vi "glueing_proc_ORIG.vi"() -> ()   [LabVIEW 2011]
panel:
  in  "spint down 2":bool
  in  "glue press 2mm":bool
  in  "spint down":bool
  in  "Start":bool
  in  "fine tuning z dw 1mm":bool
  in  "fine tuning z up 1mm":bool
  in  "goto z pos 2":bool
  in  "goto z pos":bool
  in  "goto y pos":bool
  in  "positioning done":bool
  in  "goto x pos":bool
  in  "zero Spint":bool
  out "output":string
  out "command":string
  in  "zero done":bool
  in  "zero Gluer":bool
  in  "zero x":bool
  in  "zero y":bool
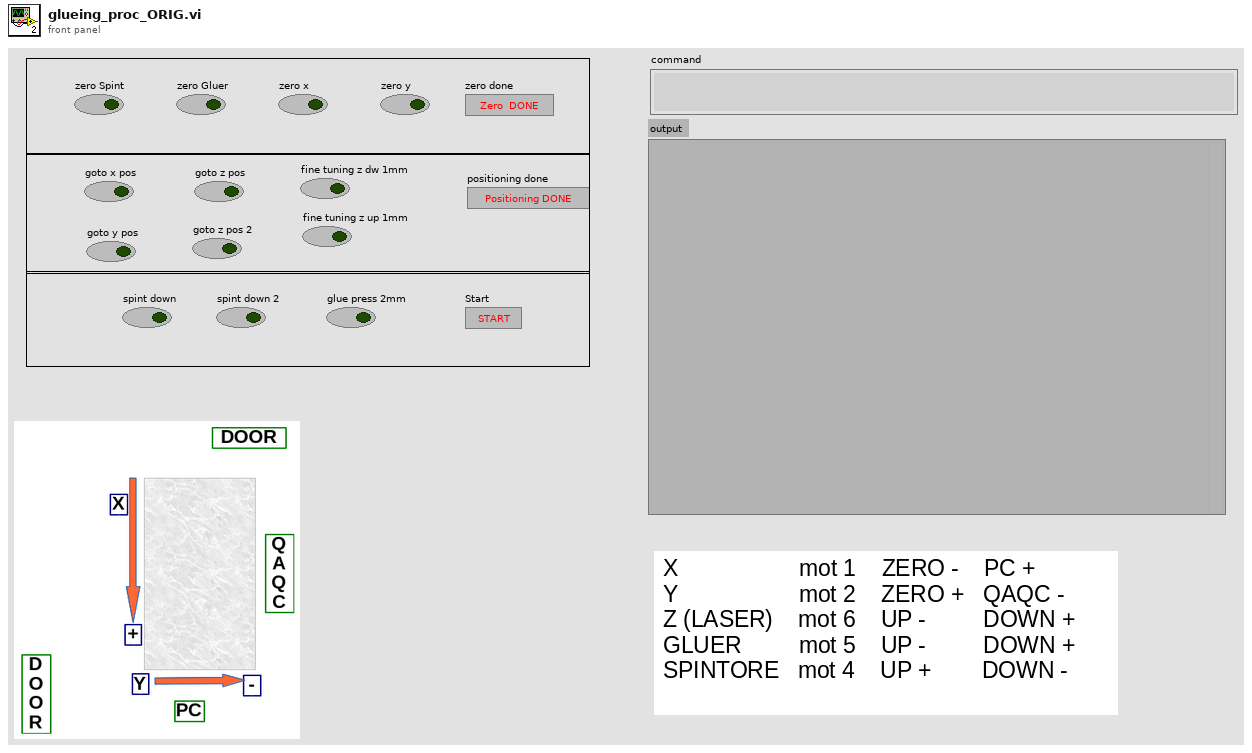
[diagram p1: front panel]
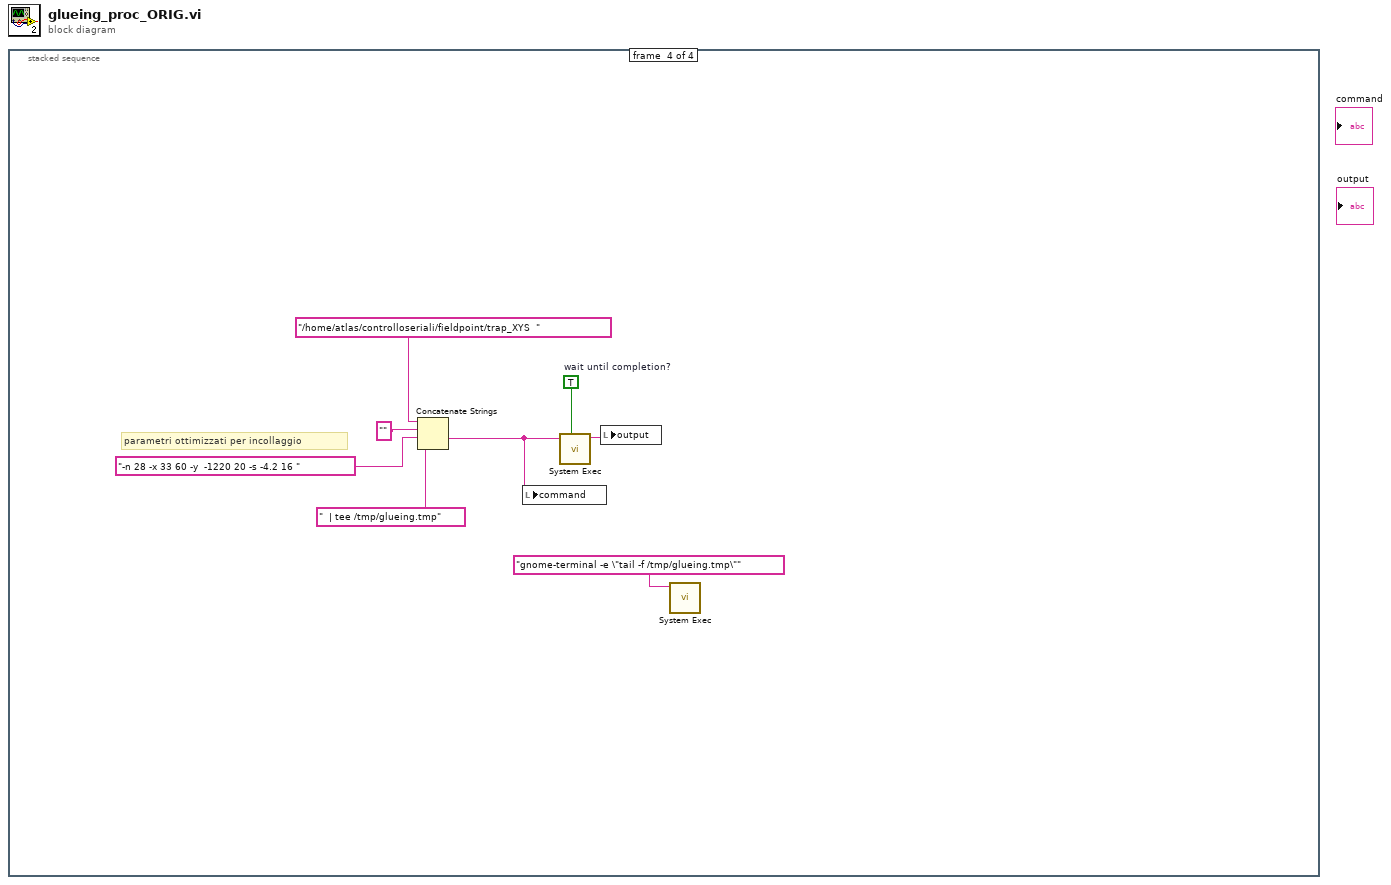
[diagram p0: block diagram]
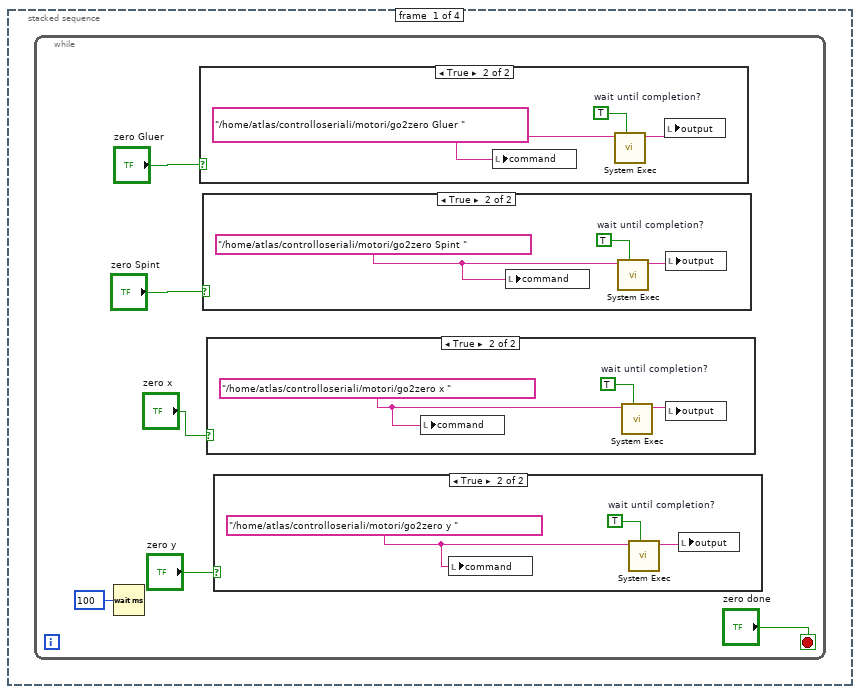
[diagram p2: hidden frame]
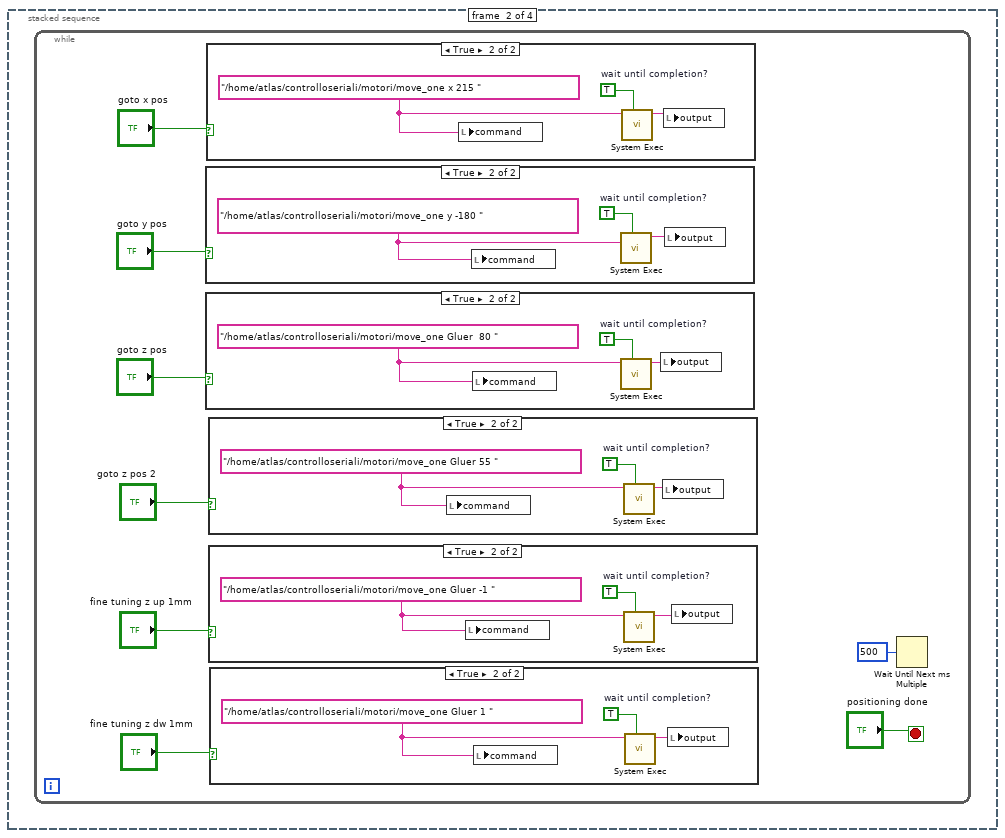
[diagram p7: hidden frame]
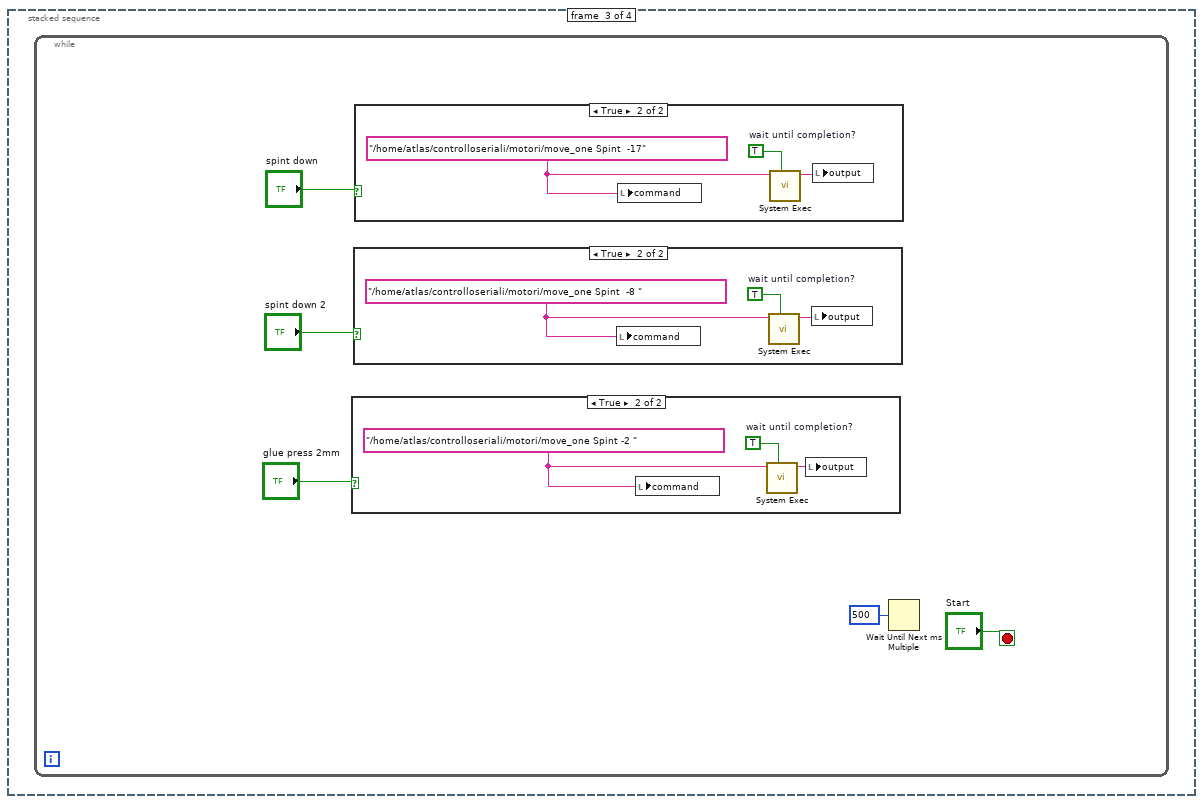
[diagram p14: hidden frame]
diagram:
  n1 = stacked-sequence {
    frame #0 {
      n2 = while {
        stop <- "zero done" stop-if-true
        n3 = Wait (ms)(milliseconds to wait=u32 100) -> ()  [unwired: 1 out]
        n4 = case shown="True" "zero Gluer" {
          frame False {
          }
          frame True {
            w17 = "/home/atlas/controlloseriali/motori/go2zero Gluer " ("string")
            w18 = TRUE  # wait until completion?
            n5 = local write "command"(w17) -> ()
            n6 = call <vilib>:"System Exec.vi"("wait until completion? (T)"=w18, "command line"=w17) -> ("standard output"=w16:string)  [unwired: 6 in, 3 out]
            n7 = local write "output"(w16) -> ()
          }
        }
        n8 = case shown="True" "zero Spint" {
          frame False {
          }
          frame True {
            w7 = "/home/atlas/controlloseriali/motori/go2zero Spint " ("string")
            w9 = TRUE  # wait until completion?
            n9 = local write "command"(w7) -> ()
            n10 = call <vilib>:"System Exec.vi"("wait until completion? (T)"=w9, "command line"=w7) -> ("standard output"=w8:string)  [unwired: 6 in, 3 out]
            n11 = local write "output"(w8) -> ()
          }
        }
        n12 = case shown="True" "zero x" {
          frame False {
          }
          frame True {
            w14 = "/home/atlas/controlloseriali/motori/go2zero x " ("string")
            w15 = TRUE  # wait until completion?
            n13 = local write "command"(w14) -> ()
            n14 = call <vilib>:"System Exec.vi"("wait until completion? (T)"=w15, "command line"=w14) -> ("standard output"=w13:string)  [unwired: 6 in, 3 out]
            n15 = local write "output"(w13) -> ()
          }
        }
        n16 = case shown="True" "zero y" {
          frame False {
          }
          frame True {
            w11 = "/home/atlas/controlloseriali/motori/go2zero y " ("string")
            w12 = TRUE  # wait until completion?
            n17 = local write "command"(w11) -> ()
            n18 = call <vilib>:"System Exec.vi"("wait until completion? (T)"=w12, "command line"=w11) -> ("standard output"=w10:string)  [unwired: 6 in, 3 out]
            n19 = local write "output"(w10) -> ()
          }
        }
      }
    }
    frame #1 {
      n20 = while {
        stop <- "positioning done" stop-if-true
        n21 = case shown="True" "goto y pos" {
          frame False {
          }
          frame True {
            w39 = "/home/atlas/controlloseriali/motori/move_one y -180 " ("string")
            w41 = TRUE  # wait until completion?
            n22 = local write "command"(w39) -> ()
            n23 = call <vilib>:"System Exec.vi"("wait until completion? (T)"=w41, "command line"=w39) -> ("standard output"=w40:string)  [unwired: 6 in, 3 out]
            n24 = local write "output"(w40) -> ()
          }
        }
        n25 = case shown="True" "goto z pos" {
          frame False {
          }
          frame True {
            w36 = "/home/atlas/controlloseriali/motori/move_one Gluer  80 " ("string")
            w38 = TRUE  # wait until completion?
            n26 = local write "command"(w36) -> ()
            n27 = call <vilib>:"System Exec.vi"("wait until completion? (T)"=w38, "command line"=w36) -> ("standard output"=w37:string)  [unwired: 6 in, 3 out]
            n28 = local write "output"(w37) -> ()
          }
        }
        n29 = case shown="True" "goto x pos" {
          frame False {
          }
          frame True {
            w42 = "/home/atlas/controlloseriali/motori/move_one x 215 " ("string")
            w44 = TRUE  # wait until completion?
            n30 = local write "command"(w42) -> ()
            n31 = call <vilib>:"System Exec.vi"("wait until completion? (T)"=w44, "command line"=w42) -> ("standard output"=w43:string)  [unwired: 6 in, 3 out]
            n32 = local write "output"(w43) -> ()
          }
        }
        n33 = case shown="True" "goto z pos 2" {
          frame False {
          }
          frame True {
            w33 = "/home/atlas/controlloseriali/motori/move_one Gluer 55 " ("string")
            w35 = TRUE  # wait until completion?
            n34 = local write "command"(w33) -> ()
            n35 = call <vilib>:"System Exec.vi"("wait until completion? (T)"=w35, "command line"=w33) -> ("standard output"=w34:string)  [unwired: 6 in, 3 out]
            n36 = local write "output"(w34) -> ()
          }
        }
        n37 = case shown="True" "fine tuning z up 1mm" {
          frame False {
          }
          frame True {
            w30 = "/home/atlas/controlloseriali/motori/move_one Gluer -1 " ("string")
            w32 = TRUE  # wait until completion?
            n38 = local write "command"(w30) -> ()
            n39 = call <vilib>:"System Exec.vi"("wait until completion? (T)"=w32, "command line"=w30) -> ("standard output"=w31:string)  [unwired: 6 in, 3 out]
            n40 = local write "output"(w31) -> ()
          }
        }
        n41 = case shown="True" "fine tuning z dw 1mm" {
          frame False {
          }
          frame True {
            w27 = "/home/atlas/controlloseriali/motori/move_one Gluer 1 " ("string")
            w29 = TRUE  # wait until completion?
            n42 = local write "command"(w27) -> ()
            n43 = call <vilib>:"System Exec.vi"("wait until completion? (T)"=w29, "command line"=w27) -> ("standard output"=w28:string)  [unwired: 6 in, 3 out]
            n44 = local write "output"(w28) -> ()
          }
        }
        n45 = Wait Until Next ms Multiple(millisecond multiple=u32 500) -> ()  [unwired: 1 out]
      }
    }
    frame #2 {
      n46 = while {
        stop <- "Start" stop-if-true
        n47 = case shown="True" "glue press 2mm" {
          frame False {
          }
          frame True {
            w54 = "/home/atlas/controlloseriali/motori/move_one Spint -2 " ("string")
            w55 = TRUE  # wait until completion?
            n48 = local write "command"(w54) -> ()
            n49 = call <vilib>:"System Exec.vi"("wait until completion? (T)"=w55, "command line"=w54) -> ("standard output"=w53:string)  [unwired: 6 in, 3 out]
            n50 = local write "output"(w53) -> ()
          }
        }
        n51 = case shown="True" "spint down 2" {
          frame False {
          }
          frame True {
            w50 = "/home/atlas/controlloseriali/motori/move_one Spint  -8 " ("string")
            w52 = TRUE  # wait until completion?
            n52 = local write "command"(w50) -> ()
            n53 = call <vilib>:"System Exec.vi"("wait until completion? (T)"=w52, "command line"=w50) -> ("standard output"=w51:string)  [unwired: 6 in, 3 out]
            n54 = local write "output"(w51) -> ()
          }
        }
        n55 = case shown="True" "spint down" {
          frame False {
          }
          frame True {
            w56 = "/home/atlas/controlloseriali/motori/move_one Spint  -17" ("string")
            w58 = TRUE  # wait until completion?
            n56 = local write "command"(w56) -> ()
            n57 = call <vilib>:"System Exec.vi"("wait until completion? (T)"=w58, "command line"=w56) -> ("standard output"=w57:string)  [unwired: 6 in, 3 out]
            n58 = local write "output"(w57) -> ()
          }
        }
        n59 = Wait Until Next ms Multiple(millisecond multiple=u32 500) -> ()  [unwired: 1 out]
      }
    }
    frame #3 {
      w66 = TRUE  # wait until completion?
      # "parametri ottimizzati per incollaggio"
      n60 = Concatenate Strings("/home/atlas/controlloseriali/fieldpoint/trap_XYS  " ("string"), "" ("string"), "-n 28 -x 33 60 -y  -1220 20 -s -4.2 16 " ("string"), "  | tee /tmp/glueing.tmp" ("string")) -> (w60:string)
      n61 = local write "command"(w60) -> ()
      n62 = call <vilib>:"System Exec.vi"("wait until completion? (T)"=w66, "command line"=w60) -> ("standard output"=w59:string)  [unwired: 6 in, 3 out]
      n63 = local write "output"(w59) -> ()
      n64 = call <vilib>:"System Exec.vi"("command line"="gnome-terminal -e \"tail -f /tmp/glueing.tmp\"" ("logwindow")) -> ()  [unwired: 7 in, 4 out]
    }
  }
